vi "Sort Image Table.vi"(3 "Images in":T2(array[cluster])) -> (1 "Images out":T1(array[cluster]))   [LabVIEW 2021, in "TSC Button Editor.lvclass"]
doc: "This VI reshapes the array of images into the display for the button editor UI.\n\n<b>Code Developed By:</b>\nTechnology Service Corporation\nwww.tsc.com/atcs\n\nDeveloper:\nDaniel Coons"
uses:
  TSC Button Editor.lvclass
  TSC Button Editor.lvclass/TSC Button Editor.ctl
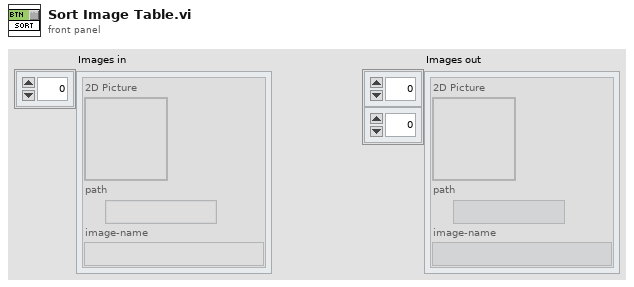
[diagram p1: front panel]
types:
  T1 = cluster{"2D Picture":picture, "path":path, "image-name":string}[][]
  T2 = cluster{"2D Picture":picture, "path":path, "image-name":string}[]
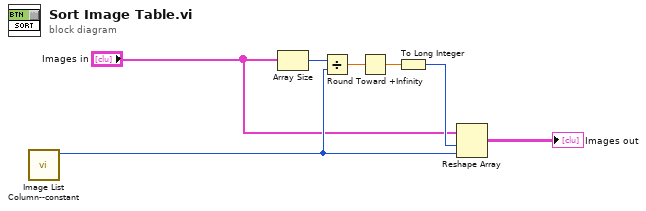
[diagram p0: block diagram]
diagram:
  n1 = call "Image List Column--constant.vi"() -> ("columns"=w3:i32)  [unwired: 11 in]
  n2 = Array Size(array="Images in") -> (size(s)=w7:i32)
  n3 = Divide(x=w7, y=w3) -> (x/y=w6:dbl)
  n4 = Round Toward +Infinity(x=w6) -> (ceil(x): smallest int >= x=w5:dbl)
  n5 = To Long Integer(number=w5) -> (32bit integer=w4:i32)
  n6 = Reshape Array "Reshape Array"("Images in", w4, w3) -> (→"Images out":T1)
